vi "Autonomous Independent.vi"() -> ()   [LabVIEW 2013]
doc: "This VI is called when autonomous begins, and will automatically be terminated when autonomous ends. You can carry out timed or sensor driven robot movement independently without needing to return to the caller."
uses:
  <vilib>/Rock Robotics/WPI/Relay/WPI_RelayValue.ctl
  Robot Global Data.vi
  <vilib>/Rock Robotics/WPI/Joystick/WPI_JoystickGetSetRefNum.vi
  <vilib>/Rock Robotics/WPI/RobotDrive/WPI_RobotDriveArcadeDrive_Standard(NoSaturation).vi
panel:
  out "Shooter":bool
  out "Current Movement, for debugging":T1 {"Y Joystick Value" scale=1.0..-1.0; "X Joystick Value" scale=-1.0..1.0}
  in  "Array of robot movements":T2(array[cluster]) {"Y Joystick Value" scale=1.0..-1.0; "X Joystick Value" scale=-1.0..1.0}
  # "Be sure to right-click and choose Data Operations>>Make Current Value default if you want to save the array values with the VI"
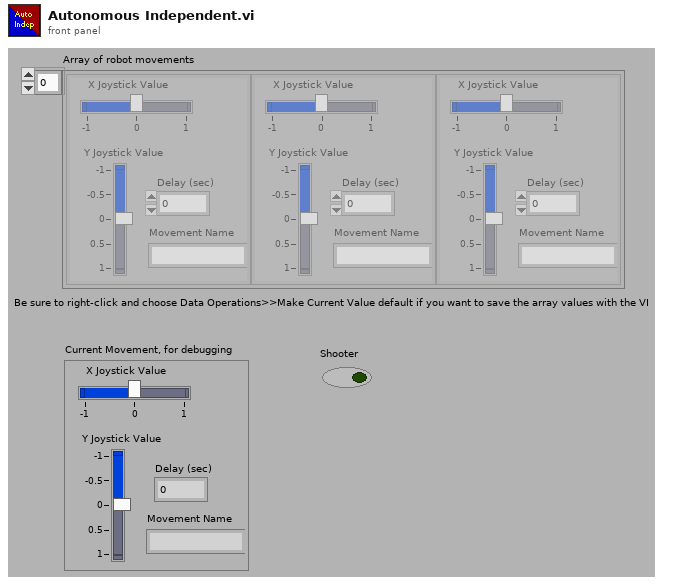
[diagram p1: front panel]
types:
  T1 = cluster{"X Joystick Value":dbl, "Y Joystick Value":dbl, "Delay (sec)":dbl, "Movement Name":string}
  T2 = cluster{"X Joystick Value":dbl, "Y Joystick Value":dbl, "Delay (sec)":dbl, "Movement Name":string}[]
  T3 = typedef "WPI_JoystickDevRef.ctl" = cluster{"Device":T4}
  T4 = typedef "WPI_JoystickDeviceEnum.ctl" = enum16{"USB 1", "USB 2", "USB 3", "USB 4", "Kinect 1", "Kinect 2"}
  T5 = cluster{"axis 1 (x)":dbl, "axis 2 (y)":dbl, "axis 3 (throttle)":dbl, "axis 4":dbl, "axis 5":dbl, "axis 6":dbl}
  T6 = typedef "WPI_RelayDevRef.ctl" = cluster{"DevStatus":errorcluster, "Relay Channel":T7, "Digital Module":T8, "Relay Direction":T9}
  T7 = typedef "FPGA_DIORelayChannel.ctl" = enum8{"Relay 1", "Relay 2", "Relay 3", "Relay 4", "Relay 5", "Relay 6", "Relay 7", "Relay 8", "Invalid"}
  T8 = typedef "FPGA_TypedefDigitalModule.ctl" = enum16{"Digital Module 1", "Digital Module 2"}
  T9 = typedef "WPI_RelayDirection.ctl" = enum16{"Both directions", "Forward only", "Reverse only"}
  T10 = typedef "WPI_RelayValue.ctl" = enum16{"Off", "On", "Forward", "Reverse"}
  T11 = typedef "WPI_MotorControlDeviceRef.ctl" = cluster{"DeviceStatus":errorcluster, "Type":enum16{"PWM", "CAN"}, "PWM":cluster{"Digital Module":T8, "PWM Channel":T12, "DeadBand":T13}, "CAN":cluster{"Device Number":u8, "Control Mode":T14, "Semaphore":T15, "Max Vout":dbl}, "Invert":bool, "TransformRef":T16, "InvTransformRef":T16}
  T12 = typedef "FPGA_DIOPWMChannel.ctl" = enum8{"PWM 1", "PWM 2", "PWM 3", "PWM 4", "PWM 5", "PWM 6", "PWM 7", "PWM 8", "PWM 9", "PWM 10", "Invalid"}
  T13 = typedef "WPI_PWMDeadband.ctl" = cluster{"Name":string, "maxPositivePwm":i32, "minPositivePwm":i32, "centerPwm":i32, "maxNegativePwm":i32, "minNegativePwm":i32, "angularRange":u16}
  T14 = typedef "WPI_CANJaguar_ControlMode.ctl" = enum8{"Percent VBus", "Current", "Speed", "Position", "Voltage"}
  T15 = typedef "Semaphore RefNum" = refnum<k1>
  T16 = typedef "WPI_PWMTransform_ConPane.ctl" = refnum<vi>
  T17 = typedef "WPI_RobotDriveDevRef.ctl" = cluster{"DevStatus":errorcluster, "Motors[]":T11[], "Square Inputs":bool, "Max Output":dbl, "Isochronous":bool}
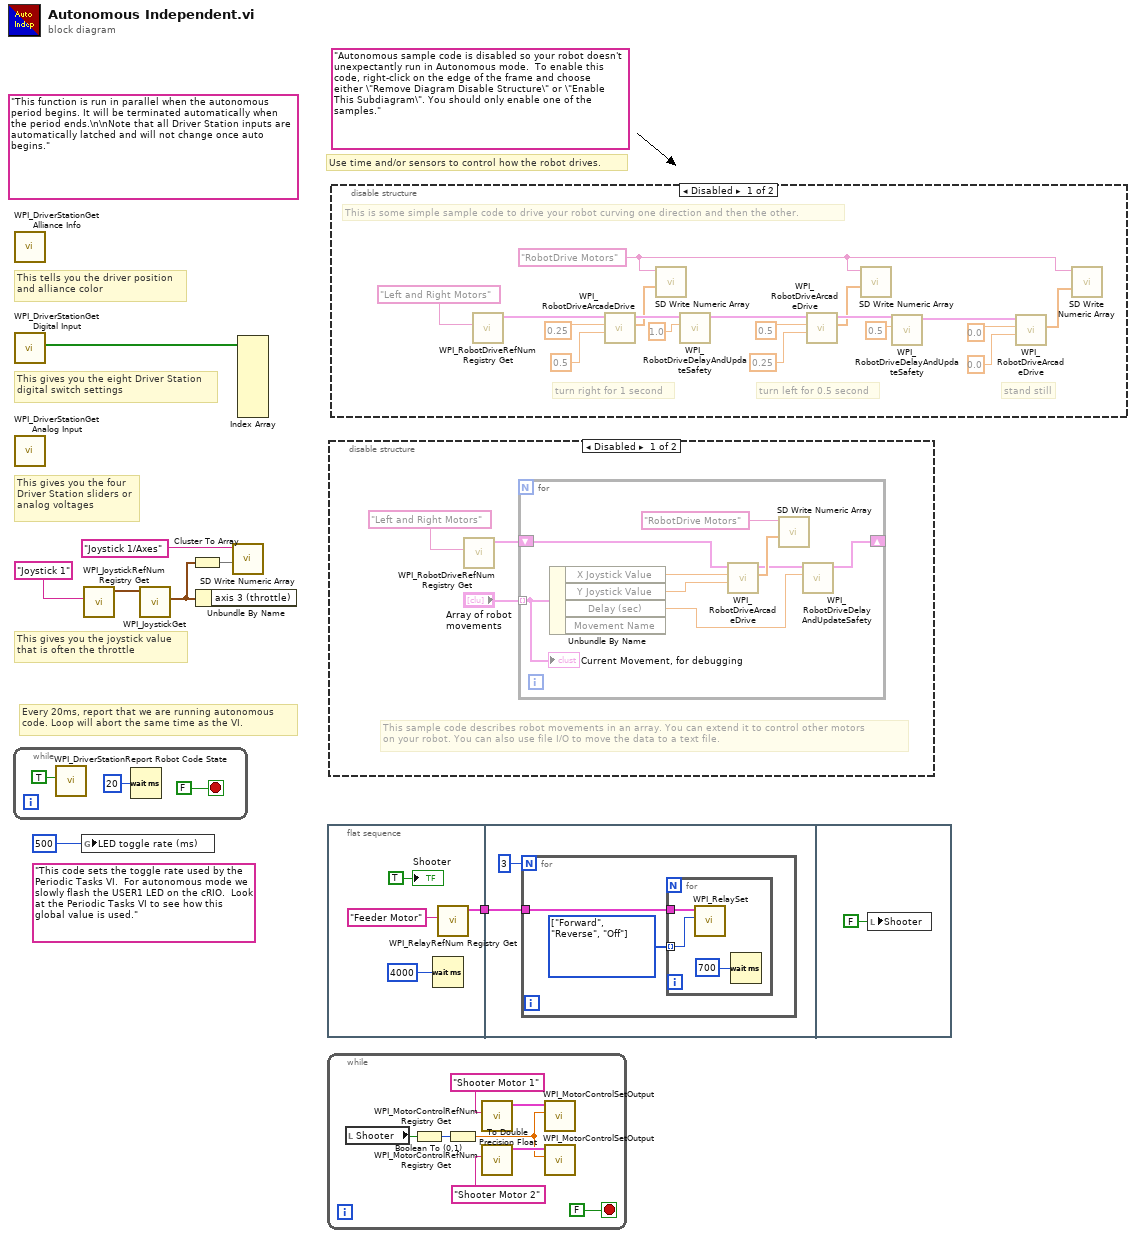
[diagram p0: block diagram]
diagram:
  (unwired) "This code sets the toggle rate used by the Periodic Tasks VI.  For autonomous mode we slowly flash the USER1 LED on the cRIO.  Look at the Periodic Tasks VI to see how this global value is used."
  (unwired) "Autonomous sample code is disabled so your robot doesn't unexpectantly run in Autonomous mode.  To enable this code, right-click on the edge of the frame and choose either \"Remove Diagram Disable Structure\" or \"Enable This Subdiagram\". You should only enable one of the samples."
  (unwired) "This function is run in parallel when the autonomous period begins. It will be terminated automatically when the period ends.\n\nNote that all Driver Station inputs are automatically latched and will not change once auto begins."
  # "Every 20ms, report that we are running autonomous\ncode. Loop will abort the same time as the VI."
  # "This gives you the joystick value\nthat is often the throttle"
  # "Use time and/or sensors to control how the robot drives."
  # "This tells you the driver position\nand alliance color"
  # "This gives you the eight Driver Station\ndigital switch settings"
  # "This gives you the four\nDriver Station sliders or\nanalog voltages"
  n1 = while {
    stop <- FALSE stop-if-true
    n2 = call <vilib>:"WPI_DriverStationReport Robot Code State.vi"("Autonomous"=TRUE) -> ()  [unwired: 10 in, 1 out]
    n3 = Wait (ms)(milliseconds to wait=u32 20) -> ()  [unwired: 1 out]
  }
  n4 = call <vilib>:"WPI_DriverStationGet Alliance Info.vi"() -> ()  [unwired: 12 out]
  n5 = call <vilib>:"WPI_DriverStationGet Digital Input.vi"() -> ("Driver Station Digital Input (1-8)"=w8:bool[])  [unwired: 11 out]
  n6 = call <vilib>:"WPI_DriverStationGet Analog Input.vi"() -> ()  [unwired: 12 out]
  n7 = global write "Robot Global Data.vi" "LED toggle rate (ms)"(u32 500 ("LED ms toggle rate")) -> ()
  n8 = call <vilib>:"WPI_JoystickRefNum Registry Get.vi"("refnum name"="Joystick 1") -> ("JoystickDevRef"=w6:T3)  [unwired: 1 in, 9 out]
  n9 = call <vilib>:"WPI_JoystickGet.vi"("JoystickDevRef"=w6) -> ("Axes"=w3:T5)  [unwired: 1 in, 5 out]
  n10 = Cluster To Array(cluster=w3) -> (array=w4:dbl[])
  n11 = Unbundle By Name(w3) -> ()  [unwired: 1 out]
  n12 = call <vilib>:"SD Write Numeric Array.vi"("Numeric Array"=w4, "Name"="Joystick 1/Axes") -> ()  [unwired: 8 in, 2 out]
  n13 = Index Array(array=w8) -> ()  [unwired: 8 in, 8 out]
  n14 = flat-sequence {
    tunnel: [w13] -> w1
    tunnel: w1 -> [w16]
    frame #0 {
      n15 = Wait (ms)(milliseconds to wait=u32 4000) -> ()  [unwired: 1 out]
      n16 = call <vilib>:"WPI_RelayRefNum Registry Get.vi"("refnum name"="Feeder Motor") -> ("RelayDevRef"=w13:T6)  [unwired: 9 in, 1 out]
      "Shooter" <- TRUE ("Shooter")
    }
    frame #1 {
      n17 = for {
        N: 3 -> [_]
        tunnel: w16 -> [w18]
        w19 = T10[] [enum."Forward", enum."Reverse", enum."Off"] items=["Off", "On", "Forward", "Reverse"]
        n18 = for {
          tunnel: w18 -> [w21]
          tunnel: w19 -> [w20] mode=indexing
          n19 = call <vilib>:"WPI_RelaySet.vi"("RelayValue"=w20, "RelayDevRef"=w21) -> ()  [unwired: 8 in, 2 out]
          n20 = Wait (ms)(milliseconds to wait=u32 700) -> ()  [unwired: 1 out]
        }
      }
    }
    frame #2 {
      n21 = local write "Shooter"(FALSE ("Shooter")) -> ()
    }
  }
  n22 = while {
    stop <- FALSE stop-if-true
    n23 = local read "Shooter"() -> (w25:bool)
    n24 = Boolean To (0,1)(Boolean=w25) -> (0, 1=w26:i16)
    n25 = To Double Precision Float(number=w26) -> (double precision float=w24:dbl)
    n26 = call <vilib>:"WPI_MotorControlRefNum Registry Get.vi"("refnum name"="Shooter Motor 1") -> ("MotorControlDevRef"=w31:T11)  [unwired: 9 in, 1 out]
    n27 = call <vilib>:"WPI_MotorControlRefNum Registry Get.vi"("refnum name"="Shooter Motor 2") -> ("MotorControlDevRef"=w30:T11)  [unwired: 9 in, 1 out]
    n28 = call <vilib>:"WPI_MotorControlSetOutput.vi"("Output"=w24, "MotorControlDevRef"=w31) -> ()  [unwired: 7 in, 3 out]
    n29 = call <vilib>:"WPI_MotorControlSetOutput.vi"("Output"=w24, "MotorControlDevRef"=w30) -> ()  [unwired: 7 in, 3 out]
  }
  n30 = disable-structure shown="Disabled" {
    frame Disabled {
      # "This sample code describes robot movements in an array. You can extend it to control other motors\non your robot. You can also use file I/O to move the data to a text file."
      n31 = call <vilib>:"WPI_RobotDriveRefNum Registry Get.vi"("refnum name"="Left and Right Motors") -> ("RobotDriveDevRef"=w33:T17)  [unwired: 1 in, 9 out]
      n32 = for {
        shift-right: [w39] -> _
        shift-left: w33 -> [w40]
        tunnel: "Array of robot movements" -> [w35] mode=indexing
        n33 = Unbundle By Name(w35) -> ("X Joystick Value"=w38:dbl, "Y Joystick Value"=w37:dbl, "Delay (sec)"=w36:dbl)  [unwired: 1 out]
        n34 = call-poly <vilib>:"WPI_RobotDriveArcadeDrive.vi"("Y axis value"=w37, "X axis value"=w38, "RobotDriveDevRef"=w40) -> ("Motor Values"=w42:dbl[], "RobotDriveDevRef"=w41:T17)  [unwired: 1 in, 6 out]
        n35 = call <vilib>:"SD Write Numeric Array.vi"("Numeric Array"=w42, "Name"="RobotDrive Motors") -> ()  [unwired: 8 in, 2 out]
        n36 = call <vilib>:"WPI_RobotDriveDelayAndUpdateSafety.vi"("Delay (s)"=w36, "RobotDriveDevRef"=w41) -> ("RobotDriveDevRef 2"=w39:T17)  [unwired: 8 in, 1 out]
        "Current Movement, for debugging" <- w35
      }
    }
    frame Enabled {
    }
  }
  n37 = disable-structure shown="Disabled" {
    frame Disabled {
      w44 = "RobotDrive Motors" ("Name")
      # "This is some simple sample code to drive your robot curving one direction and then the other."
      # "stand still"
      # "turn left for 0.5 second"
      # "turn right for 1 second"
      n38 = call <vilib>:"WPI_RobotDriveRefNum Registry Get.vi"("refnum name"="Left and Right Motors") -> ("RobotDriveDevRef"=w48:T17)  [unwired: 1 in, 9 out]
      n39 = call-poly <vilib>:"WPI_RobotDriveArcadeDrive.vi"("Y axis value"=0.5 ("X axis value"), "X axis value"=0.25, "RobotDriveDevRef"=w48) -> ("Motor Values"=w47:dbl[], "RobotDriveDevRef"=w55:T17)  [unwired: 1 in, 6 out]
      n40 = call <vilib>:"SD Write Numeric Array.vi"("Numeric Array"=w47, "Name"=w44) -> ()  [unwired: 8 in, 2 out]
      n41 = call <vilib>:"WPI_RobotDriveDelayAndUpdateSafety.vi"("Delay (s)"=1.0, "RobotDriveDevRef"=w55) -> ("RobotDriveDevRef 2"=w54:T17)  [unwired: 8 in, 1 out]
      n42 = call-poly <vilib>:"WPI_RobotDriveArcadeDrive.vi"("Y axis value"=0.25 ("X axis value"), "X axis value"=0.5, "RobotDriveDevRef"=w54) -> ("Motor Values"=w46:dbl[], "RobotDriveDevRef"=w53:T17)  [unwired: 1 in, 6 out]
      n43 = call <vilib>:"SD Write Numeric Array.vi"("Numeric Array"=w46, "Name"=w44) -> ()  [unwired: 8 in, 2 out]
      n44 = call <vilib>:"WPI_RobotDriveDelayAndUpdateSafety.vi"("Delay (s)"=0.5, "RobotDriveDevRef"=w53) -> ("RobotDriveDevRef 2"=w52:T17)  [unwired: 8 in, 1 out]
      n45 = call-poly <vilib>:"WPI_RobotDriveArcadeDrive.vi"("Y axis value"=0.0 ("X axis value"), "X axis value"=0.0, "RobotDriveDevRef"=w52) -> ("Motor Values"=w45:dbl[])  [unwired: 1 in, 7 out]
      n46 = call <vilib>:"SD Write Numeric Array.vi"("Numeric Array"=w45, "Name"=w44) -> ()  [unwired: 8 in, 2 out]
    }
    frame Enabled {
    }
  }
